vi "reciver.vi"() -> ()   [LabVIEW 2017]
uses:
  <vilib>/addons/Modulation/Analog/support/mod_Set Error Source.vi
  <vilib>/addons/Modulation/Analog/support/Validators/mod_Fractional Resample Validate.vi
  <vilib>/addons/Modulation/Analog/support/Validators/mod_Check Flush State.vi
  <vilib>/addons/Modulation/Analog/support/mod_FractionalResampler.vi
  <vilib>/addons/Modulation/Analog/support/mod_Integer Rate Interpolation.vi
  <vilib>/addons/Modulation/Analog/support/Validators/mod_Validate Complex Waveform.vi
  <vilib>/addons/Modulation/Analog/support/mod_PerformResampling.vi
  <vilib>/addons/Modulation/Analog/support/Validators/mod_WFErrorHandler.vi
  <vilib>/addons/Modulation/Digital/General/MT Generate MSK System Parameters.vi
  <vilib>/addons/Modulation/Digital/Support/Common/Validators/mod_Generate Filter Coefficients Validate.vi
  <vilib>/addons/Modulation/Digital/General/subVIs/mod_Generate Filter Coefficients.vi
  <instrlib>/niUSRP/niUSRP Fetch Rx Data (CDB Cluster).vi
  <vilib>/Utility/error.llb/Error Cluster From Error Code.vi
  <vilib>/addons/Modulation/Analog/support/mod_Resampling Factors.vi
  <vilib>/addons/Modulation/Analog/support/mod_ResamplingFilter.vi
  <vilib>/addons/Modulation/Analog/support/mod_Generate Integer Interpolation Filter.vi
  <vilib>/addons/Modulation/niDMT.lvlib
  <vilib>/addons/Modulation/niAMT.lvlib
panel:
  out "Dmodulation constaltion":T1(graph)
  in  "number of samples":i64=1000
  out "ERROR OUT":errorcluster
  in  "ERROR iN":errorcluster
  in  "stop":bool
  out "output signal":i8[](graph)
  out "Filter shape":dbl[](graph)
  in  "simpling rate":dbl
  in  "filter length (symbols)":i32=8
  in  "active antenna":string
  out "coerced gain":dbl format="%#_6f"
  out "coerced carrier frequency":dbl=100000.0 format="%#_6p"
  out "coerced IQ rate":dbl=100000.0 format="%#_6p"
  in  "gain":dbl format="%#_6f"
  in  "carrier frequency":dbl=100000.0 format="%#_6p"
  in  "IQ rate":dbl=100000.0 format="%#_6p"
  in  "Boolean":bool
  in  "device names":refnum<k15>
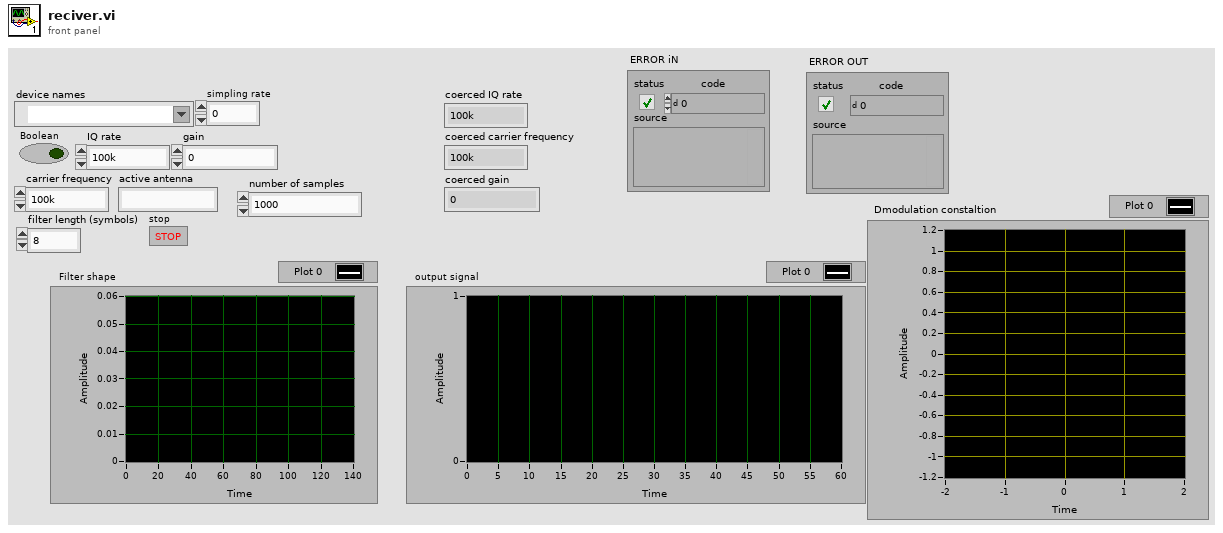
[diagram p1: front panel]
types:
  T1 = cluster{"constellation":dbl[], "oversampled data":dbl[]}[]
  T2 = enum16{"none", "Raised Cosine", "Root Raised Cos", "Gaussian"}
  T3 = enum16{"FSK", "PSK", "QAM", "MSK", "PAM", "ASK", "CPM"}
  T4 = cluster{"differential encoding enable":enum16{"disable", "enable"}, "samples per symbol (16)":i32}
  T5 = typedef "niAMT.lvlib/Complex Data Waveform.ctl" = cluster{"t0":dbl, "dt":dbl, "Y":cdb[]}
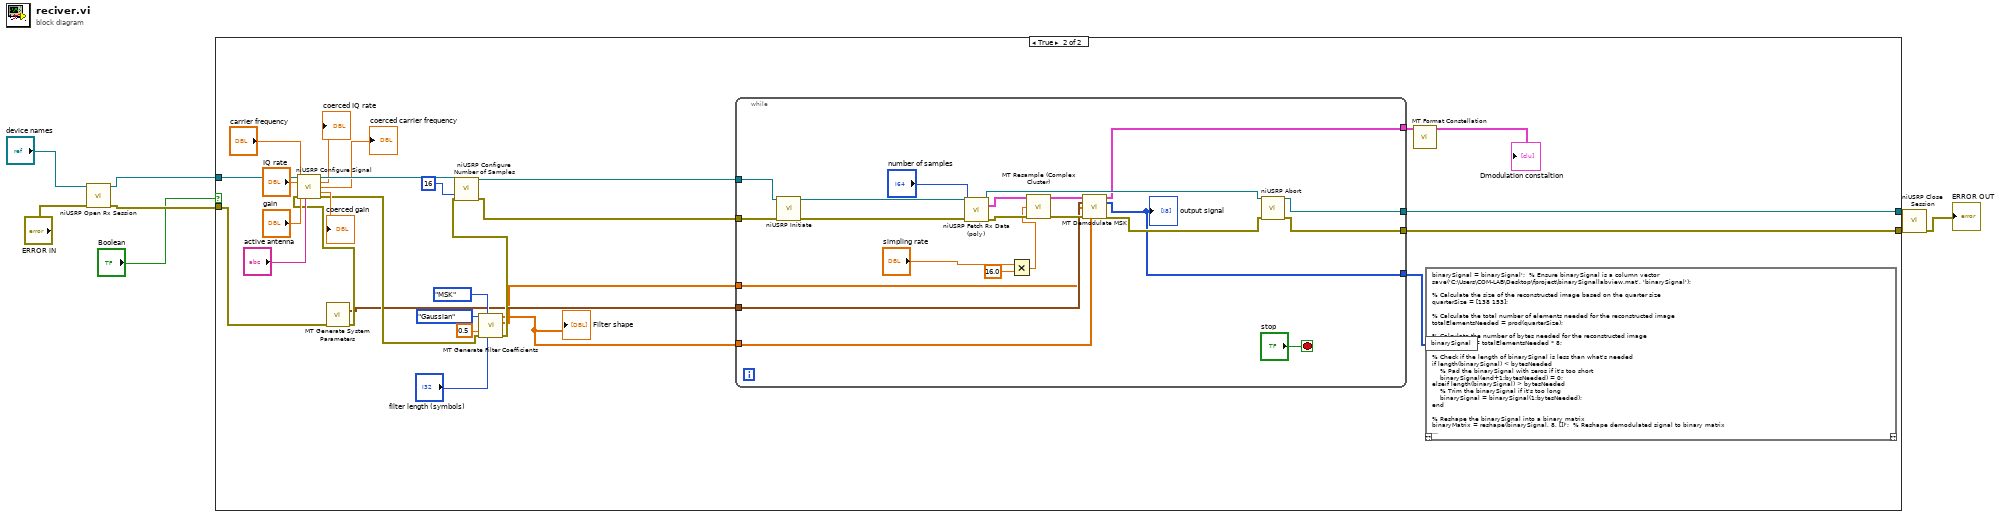
[diagram p0: block diagram]
diagram:
  n1 = call <instrlib>:"niUSRP Open Rx Session.vi"("device names"="device names", "error in (no error)"="ERROR iN") -> ("session handle out"=w8:refnum<k15>, "error out"=w7:errorcluster)  [unwired: 12 in]
  n2 = case shown="True" "Boolean" {
    tunnel: w8 -> [_ w36]
    tunnel: w7 -> [_ w24]
    tunnel: [_ w14] -> w4
    tunnel: [_ w13] -> w3
    frame False {
    }
    frame True {
      n3 = call-poly <vilib>:"MT Generate System Parameters.vi"("error in (no error)"=w24) -> ("MSK system parameters"=w17:T4, "error out"=w23:errorcluster)  [unwired: 12 in, 1 out]
      n4 = call <instrlib>:"niUSRP Configure Signal.vi"("session handle"=w36, "IQ rate"="IQ rate", "carrier frequency"="carrier frequency", "gain"="gain", "error in (no error)"=w23, "active antenna"="active antenna") -> ("session handle out"=w35:refnum<k15>, "coerced IQ rate"=→"coerced IQ rate":dbl, "coerced carrier frequency"=→"coerced carrier frequency":dbl, "coerced gain"=→"coerced gain":dbl, "error out"=w19:errorcluster)  [unwired: 5 in]
      n5 = call <vilib>:"MT Generate Filter Coefficients.vi"("pulse shaping filter (none)"=T2."Gaussian", "modulation type"=T3."MSK", "filter parameter"=0.5, "error in (no error)"=w19, "filter length (symbols)"="filter length (symbols)") -> ("pulse shaping filter coefficients"=w15:dbl[], "matched filter coefficients"=w16:dbl[], "error out"=w18:errorcluster)  [unwired: 8 in]
      "Filter shape" <- w15
      n6 = call <instrlib>:"niUSRP Configure Number of Samples.vi"("session handle"=w35, "number of samples"=i64 16, "error in (no error)"=w18) -> ("session handle out"=w33:refnum<k15>, "error out"=w34:errorcluster)  [unwired: 11 in]
      n7 = while {
        tunnel: w34 -> [w58]
        tunnel: w33 -> [w57]
        tunnel: w17 -> [w47]
        tunnel: w16 -> [w46]
        tunnel: w15 -> [w45]
        tunnel: [w42] -> w14
        tunnel: [w41] -> w13
        tunnel: [w38] -> w11
        tunnel: [w37] -> w10
        stop <- "stop" stop-if-true
        n8 = call <instrlib>:"niUSRP Initiate.vi"("session handle"=w57, "error in (no error)"=w58) -> ("session handle out"=w55:refnum<k15>, "error out"=w56:errorcluster)  [unwired: 12 in]
        n9 = call-poly <instrlib>:"niUSRP Fetch Rx Data (poly).vi"("session handle"=w55, "number of samples"="number of samples", "error in (no error)"=w56) -> ("session handle out"=w44:refnum<k15>, "data"=w54:cluster{"t0":dbl, "dt":dbl, "Y":cdb[]}, "error out"=w53:errorcluster)  [unwired: 9 in, 1 out]
        n10 = Multiply(x="simpling rate", y=16.0) -> (x*y=w48:dbl)
        n11 = call <vilib>:"MT Resample (Complex Cluster).vi"("input complex waveform"=w54, "desired sample rate (Hz)"=w48, "error in (no error)"=w53) -> ("output complex waveform"=w51:T5, "error out"=w52:errorcluster)  [unwired: 11 in]
        n12 = call <vilib>:"MT Demodulate MSK.vi"("input complex waveform"=w51, "MSK system parameters"=w47, "matched filter coefficients"=w46, "error in (no error)"=w52, "pulse shaping filter coefficients"=w45) -> ("recovered complex waveform"=w37:T5, "output bit stream"=w38:i8[], "error out"=w43:errorcluster)  [unwired: 5 in, 3 out]
        "output signal" <- w38
        n13 = call <instrlib>:"niUSRP Abort.vi"("session handle"=w44, "error in (no error)"=w43) -> ("session handle out"=w41:refnum<k15>, "error out"=w42:errorcluster)  [unwired: 12 in]
      }
      n14 = call <vilib>:"MT Format Constellation.vi"("waveform"=w10) -> ("constellation graph"=→"Dmodulation constaltion":T1)  [unwired: 13 in, 1 out]
      n15 = script code="binarySignal = binarySignal';  % Ensure binarySignal is a column vector\nsave('C:\\Users\\COM-LAB\\Desktop\\fproject\\binarySignallabview.mat', 'binarySignal');\n\n% Calculate the size of the reconstructed image based on the quarter size\nquarterSize = [138 153];\n\n% Calculate the total number of elements needed for the reconstructed image\ntotalElementsNeeded = prod(quarterSize);\n\n% Calculate the number of bytes needed for the reconstructed image\nbytesNeeded = totalElementsNeeded * 8;\n\n% Check if the length of binarySignal is less than what's needed\nif length(binarySignal) < bytesNeeded\n    % Pad the binarySignal with zeros if it's too short\n    binarySignal(end+1:bytesNeeded) = 0;\nelseif length(binarySignal) > bytesNeeded\n    % Trim the binarySignal if it's too long\n    binarySignal = binarySignal(1:bytesNeeded);\nend\n\n% Reshape the binarySignal into a binary matrix\nbinaryMatrix = reshape(binarySignal, 8, [])';  % Reshape demodulated signal to binary matrix\n\n% Convert binary values to decimal to get pixel values\ndecimalMatrix = bi2de(binaryMatrix);  \n\n% Normalize the pixel values to the range [0, 255]\nminVal = double(min(decimalMatrix));\nmaxVal = double(max(decimalMatrix));\nnormalizedDecimalMatrix = (double(decimalMatrix) - minVal) / (maxVal - minVal) * 255;\n\n% Reshape normalized decimal matrix to quarter image size\n% Ensure the total number of elements matches the required size\nreconstructedImage = reshape(normalizedDecimalMatrix(1:totalElementsNeeded), quarterSize);\n\n% Convert to uint8 for image display\nreconstructedQuarterImage = uint8(reconstructedImage);\n\n% Save the reconstructed quarter image\nimwrite(reconstructedQuarterImage, 'C:\\Users\\COM-LAB\\Desktop\\fproject\\reconstructed_image_labview.png');"("binarySignal"=w11) -> ()  [unwired: 1 in, 1 out]
    }
  }
  n16 = call <instrlib>:"niUSRP Close Session.vi"("session handle"=w3, "error in (no error)"=w4) -> ("error out"=→"ERROR OUT":errorcluster)  [unwired: 13 in]
